vi "Write.vi"(8 "error in (no error)":errorcluster, 10 "Statement":T1={"timestamp"=timestamp(0 s since 1904-01-01), "level"=enum."INFO", "sourceTag"="", "originVI"="", "message"=""}, 11 "FileAppender in":refnum<class "FileAppender.lvclass">) -> (0 "error out":errorcluster, 3 "FileAppender out":refnum<class "FileAppender.lvclass">)   [LabVIEW 2026, in "Lumberjack.lvlib" / "FileAppender.lvclass"]
doc: "Deliver one accepted Statement to the sink. Called by HandleStatement after the statement passes the appender threshold and filter. Receives the structured Statement (not a formatted string): text sinks format via their own Layout here; the relay forwards or enqueues the Statement object. Abstract. DD, must override."
uses:
  FileAppender.lvclass
  TypeDefs/Statement.ctl
  TypeDefs/Severity.ctl
  FileAppender.lvclass/FileAppender.ctl
  Layouts/Layout.lvclass/Layout.lvclass
  Lumberjack.lvlib
  Appender.lvclass/Appender.lvclass
panel:
  out "path":path
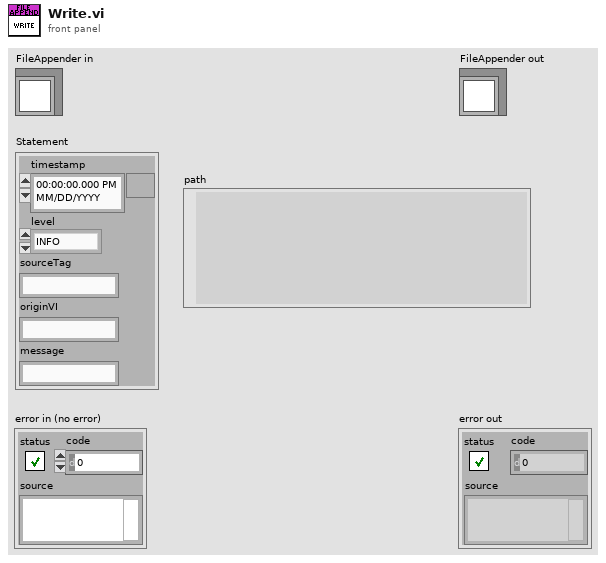
[diagram p1: front panel]
types:
  T1 = typedef "Lumberjack.lvlib/Statement.ctl" = cluster{"timestamp":timestamp, "level":T2, "sourceTag":string, "originVI":string, "message":string}
  T2 = typedef "Lumberjack.lvlib/Severity.ctl" = enum16{"OFF", "FATAL", "ERROR", "WARN", "INFO", "DEBUG", "TRACE", "ALL"}
  T3 = typedef "Lumberjack.lvlib/FileConfig.ctl" = cluster{"rootFolder":path, "maxFileSize":i64, "maxFileCount":i32, "baseName":string, "extension":string, "delimiter":string, "calendarFolderTree":bool}
  T4 = typedef "Lumberjack.lvlib/AppenderConfig.ctl" = cluster{"id":string, "threshold":T2, "filter":T5, "queueBound":i32, "dropPolicy":T7, "useUTC":bool}
  T5 = typedef "Lumberjack.lvlib/Filter.ctl" = cluster{"mode":T6, "levelMin":T2, "levelMax":T2, "tagPrefix":string}
  T6 = typedef "Lumberjack.lvlib/FilterMode.ctl" = enum16{"Mirror", "Routed"}
  T7 = typedef "Lumberjack.lvlib/DropPolicy.ctl" = enum16{"DropOldest", "DropNewest", "LevelAware"}
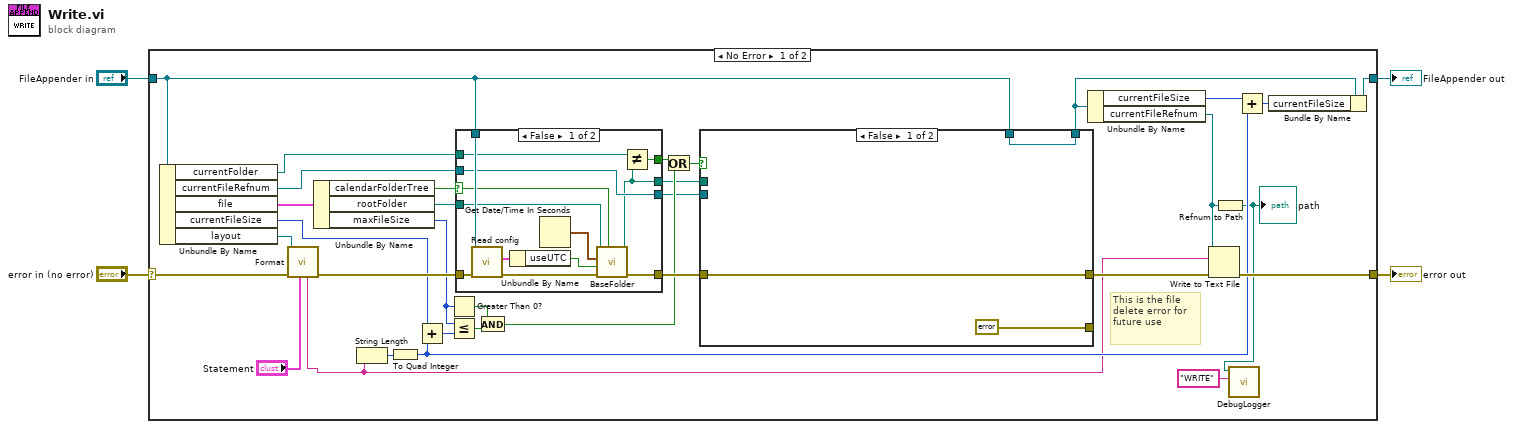
[diagram p0: block diagram]
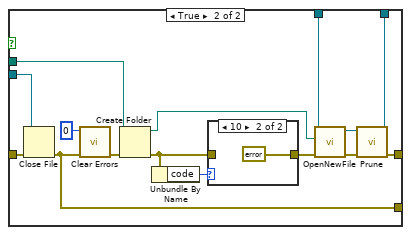
[diagram p2: hidden frame]
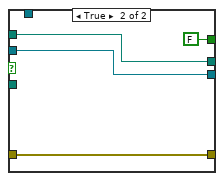
[diagram p4: hidden frame]
diagram:
  n1 = case shown="No Error" "error in (no error)" {
    selector: "error in (no error)" -> [w36 w75]
    tunnel: "FileAppender in" -> [w16 w76]
    tunnel: [w14 w75] -> w2
    tunnel: [w12 w76] -> w1
    frame No Error {
      # "This is the file delete error for future use"
      n2 = Unbundle By Name(w16) -> ("currentFolder"=w18:path, "currentFileRefnum"=w17:refnum<file>, "file"=w25:T3, "currentFileSize"=w20:i64, "layout"=w21:refnum<class "Layout.lvclass">)
      n3 = call-dynamic "Format.vi"("Statement"="Statement", "error in (no error)"=w36, "Layout in"=w21) -> ("error out"=w34:errorcluster, "FormattedLine"=w8:string)  [unwired: 6 in, 1 out]
      n4 = Unbundle By Name(w25) -> ("calendarFolderTree"=w24:bool, "rootFolder"=w23:path, "maxFileSize"=w22:i64)
      n5 = String Length(string=w8) -> (length=w35:i32)
      n6 = To Quad Integer(1:w35) -> (0:w10:i64)
      n7 = Add(x=w20, y=w10) -> (x+y=w33:i64)
      n8 = Greater Than 0?(x=w22) -> (x > 0?=w32:bool)
      n9 = Less Or Equal?(x=w22, y=w33) -> (x <= y?=w31:bool)
      n10 = case shown="False" w24 {
        selector: w24 -> [w65 _]
        tunnel: w16 -> [w70 _]
        tunnel: w23 -> [w64 _]
        tunnel: w34 -> [w63 w74]
        tunnel: [w62 w74] -> w30
        tunnel: w18 -> [w58 w71]
        tunnel: [w61 FALSE] -> w29
        tunnel: [w60 w72] -> w26
        tunnel: w17 -> [w60 w72]
        tunnel: [w59 w71] -> w19
        frame False {
          n11 = call "Read config.vi"("error in (no error)"=w63, "Appender in"=w70) -> ("error out"=w67:errorcluster, "AppenderConfig"=w69:T4)  [unwired: 7 in, 1 out]
          n12 = Unbundle By Name(w69) -> ("useUTC"=w66:bool)
          n13 = Get Date/Time In Seconds() -> (seconds since 1Jan1904=w68:timestamp)
          n14 = call "BaseFolder.vi"("calendarFolderTree"=w65, "error in (no error)"=w67, "useUTC"=w66, "Timestamp"=w68, "RootFolder"=w64) -> ("error out"=w62:errorcluster, "Folder"=w59:path)  [unwired: 5 in]
          n15 = Not Equal?(x=w58, y=w59) -> (x != y?=w61:bool)
        }
        frame True {
        }
      }
      n16 = And(x=w32, y=w31) -> (x .and. y?=w28:bool)
      n17 = Or(x=w29, y=w28) -> (x .or. y?=w27:bool)
      n18 = case shown="False" w27 {
        tunnel: w30 -> [w39 w55]
        tunnel: w26 -> [_ w54]
        tunnel: [errorcluster {"status"=FALSE, "code"=0, "source"=""} ("error out") w51] -> _
        tunnel: w19 -> [_ w46]
        tunnel: w16 -> [w38 w47]
        tunnel: [w39 w42] -> w15
        tunnel: [w38 w41] -> w13
        frame False {
        }
        frame True {
          n19 = Close File(refnum=w54, error in=w55) -> (error out=w51:errorcluster)  [unwired: 1 out]
          n20 = call <vilib>:"Clear Errors.vi"("error in (no error)"=w51, "specific error code to clear (0: all)"=0) -> ("error out"=w50:errorcluster)  [unwired: 4 in, 1 out]
          n21 = Create Folder(path (use dialog)=w46, error in=w50) -> (created path=w45:path, error out=w53:errorcluster)  [unwired: 1 in, 1 out]
          n22 = Unbundle By Name(w53) -> ("code"=w52:i32)
          n23 = case shown="10" w52 {
            tunnel: w53 -> [w56 _]
            tunnel: [w56 errorcluster {"status"=FALSE, "code"=0, "source"=""} ("error out")] -> w48
            frame Default {
            }
            frame 10 {
            }
          }
          n24 = call "OpenNewFile.vi"("error in (no error)"=w48, "targetFolder"=w45, "FileAppender in"=w47) -> ("error out"=w43:errorcluster, "FileAppender out"=w44:refnum<class "FileAppender.lvclass">)  [unwired: 7 in]
          n25 = call "Prune.vi"("error in (no error)"=w43, "FileAppender in"=w44) -> ("error out"=w42:errorcluster, "FileAppender out"=w41:refnum<class "FileAppender.lvclass">)  [unwired: 8 in]
        }
      }
      n26 = Unbundle By Name(w13) -> ("currentFileSize"=w11:i64, "currentFileRefnum"=w7:refnum<file>)
      n27 = Write to Text File(file (use dialog)=w7, text=w8, error in=w15) -> (error out=w14:errorcluster)  [unwired: 1 in, 2 out]
      n28 = Refnum to Path(1:w7) -> (0:w6:path)
      "path" <- w6
      n29 = call "DebugLogger.vi"("Message"="WRITE", "Path"=w6) -> ()  [unwired: 9 in, 1 out]
      n30 = Add(x=w11, y=w10) -> (x+y=w9:i64)
      n31 = Bundle By Name(cluster=w13, "currentFileSize"=w9) -> (w12:refnum<class "FileAppender.lvclass">)
    }
    frame Error {
    }
  }
  "error out" <- w2
  "FileAppender out" <- w1
